vi "delete cruve.vi"() -> ()   [LabVIEW 2019]
panel:
  in  "string":string
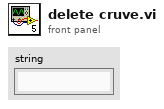
[diagram p1: front panel]
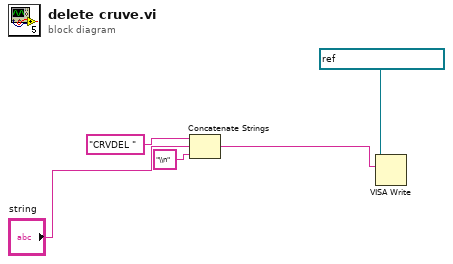
[diagram p0: block diagram]
diagram:
  n1 = Concatenate Strings("CRVDEL " ("string"), "string", "\\n" ("string")) -> (w2:string)
  n2 = VISA Write(VISA resource name=refnum<visa-resource-name> "GPIB1::12::INSTR", write buffer=w2) -> ()  [unwired: 1 in, 3 out]
